vi "InitializeFile_useVariant.vi"(4 "Digitizer Info":T2, 5 "QDC Info":T2, 6 "TDC Info":T2, 7 "Scaler Info":T2, 8 "error in":errorcluster, 9 "Trigger Bit Descriptions":string[](array[string]), 10 "Thermocouple Location":string[](array[string]), 11 "File Path":path) -> (0 "error out":errorcluster, 3 "File Handle":T1 format="%.0x")   [LabVIEW 2014]
uses:
  <vilib>/addons/h5labview2/base/hid_t.ctl
  <vilib>/addons/h5labview2/file/H5Fmode.ctl
  DatasetNames.vi
  <vilib>/addons/h5labview2/base/lib_path.vi
  <vilib>/addons/h5labview2/base/H5Equery.vi
  <vilib>/addons/h5labview2/attrib/H5Awrite.llb/H5Awrite.xnode
  <vilib>/addons/h5labview2/file/H5F.lvlib
  <vilib>/addons/h5labview2/group/H5G.lvlib
  <vilib>/addons/h5labview2/dataset/H5D.lvlib
  <vilib>/addons/h5labview2/attrib/H5A.lvlib
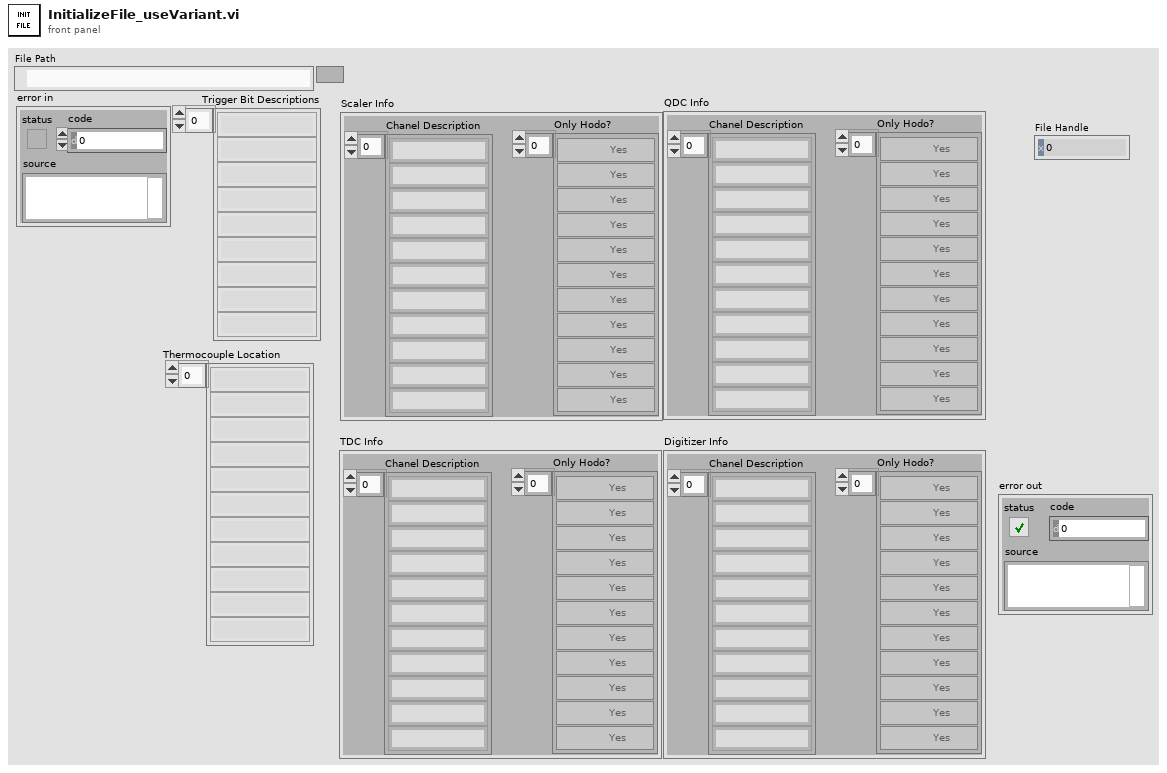
[diagram p1: front panel]
types:
  T1 = typedef "hid_t.ctl" = i32
  T2 = cluster{"Chanel Description":string[], "Only Hodo?":bool[]}
  T3 = typedef "H5F.lvlib/H5Fmode.ctl" = enum16{"read-only", "read-write", "overwrite", "create new", "open or create"}
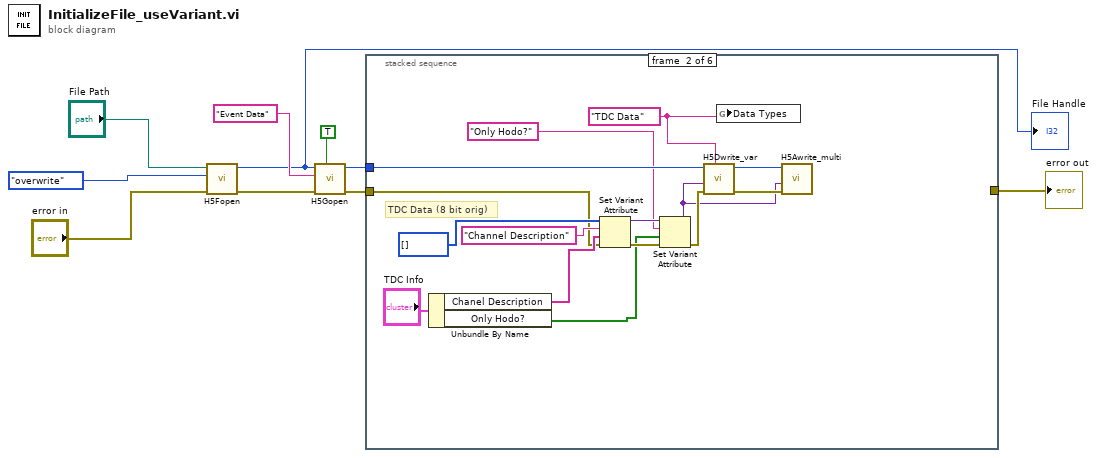
[diagram p0: block diagram]
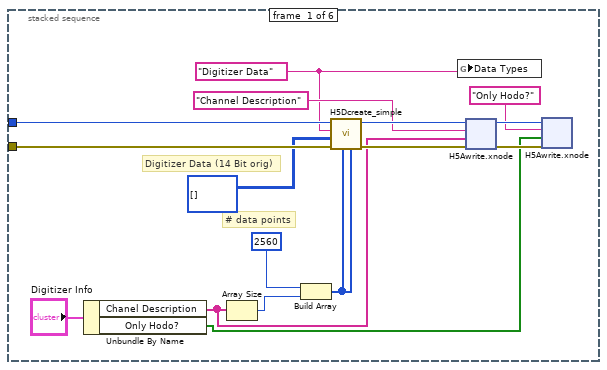
[diagram p2: hidden frame]
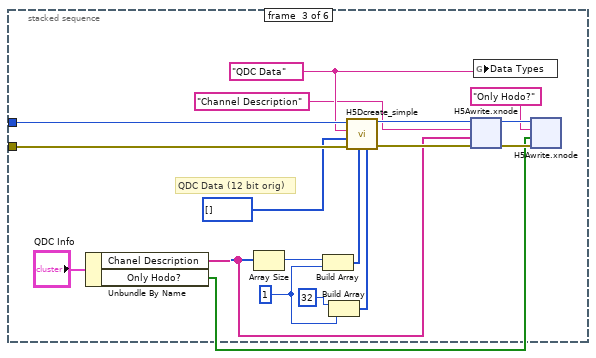
[diagram p3: hidden frame]
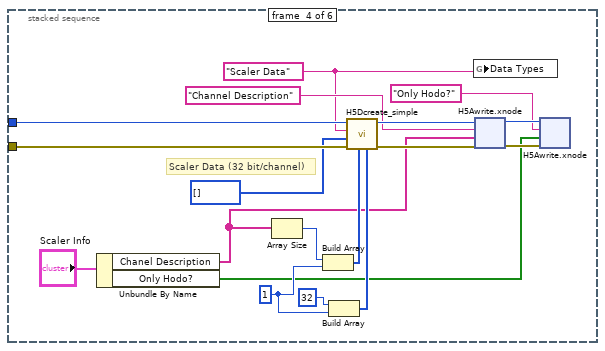
[diagram p4: hidden frame]
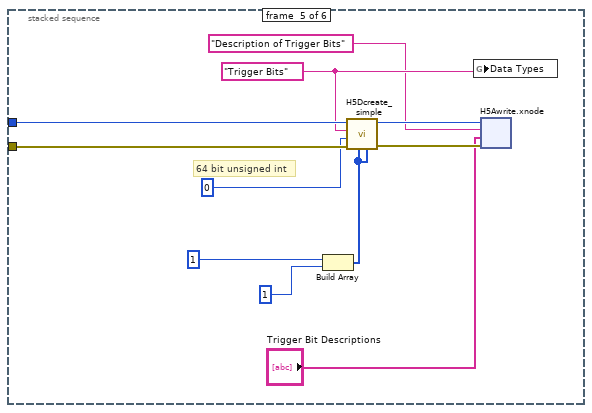
[diagram p5: hidden frame]
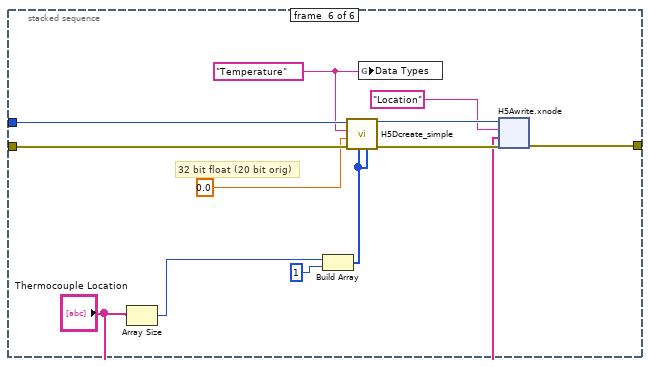
[diagram p6: hidden frame]
diagram:
  n1 = call <vilib>:"H5Fopen.vi"("error in (no error)"="error in", "mode (read-only)"=H5Fmode."overwrite", "path"="File Path") -> ("error out"=w7:errorcluster, "ref out"=w2:T1)  [unwired: 7 in]
  "File Handle" <- w2
  n2 = call <vilib>:"H5Gopen.vi"("create? (F)"=TRUE, "error in (no error)"=w7, "name"="Event Data", "ref in"=w2) -> ("error out"=w4:errorcluster, "group out"=w5:T1)  [unwired: 6 in]
  n3 = stacked-sequence {
    tunnel: w5 -> [w26 w77 w94 w148 w195 w225]
    tunnel: w4 -> [w25 w69 w95 w149 w196 w226]
    tunnel: [_ _ _ _ _ w219] -> w3
    frame #0 {
      w13 = "Digitizer Data" ("Combo Box")
      # "Digitizer Data (14 Bit orig)"
      # "# data points"
      n4 = Unbundle By Name("Digitizer Info") -> ("Chanel Description"=w16:string[], "Only Hodo?"=w11:bool[])
      n5 = Array Size(array=w16) -> (size(s)=w20:i32)
      n6 = Build Array(2560, w20) -> (w22:i32[])
      n7 = call <vilib>:"H5Dcreate_simple.vi"("max size"=w22, "initial size"=w22, "error in (no error)"=w25, "type in"=i16[][] [] ("Digitizer Data (14 Bit orig)"), "name"=w13, "ref in"=w26) -> ("error out"=w19:errorcluster, "dset out"=w18:T1)  [unwired: 4 in]
      n8 = global write "DatasetNames.vi" "Data Types"(w13) -> ()
      n9 = xnode "H5Awrite.xnode"("error in (no error)"=w19, "data"=w16, "attrib name"="Channel Description", "ref in"=w18) -> ("error out"=w15:errorcluster, "ref out"=w14:i32)  [unwired: 3 in, 1 out]
      n10 = xnode "H5Awrite.xnode"("error in (no error)"=w15, "data"=w11, "attrib name"="Only Hodo?", "ref in"=w14) -> ()  [unwired: 3 in, 3 out]
    }
    frame #1 {
      w75 = "TDC Data" ("Combo Box")
      # "TDC Data (8 bit orig)"
      n11 = Unbundle By Name("TDC Info") -> ("Chanel Description"=w72:string[], "Only Hodo?"=w67:bool[])
      n12 = Set Variant Attribute(Variant=i16[] [] ("TDC Data (8 bit orig)"), name="Channel Description" ("attrib name"), value=w72, error in=w69) -> (Variant out=w70:variant, error out=w71:errorcluster)  [unwired: 1 out]
      n13 = Set Variant Attribute(Variant=w70, name="Only Hodo?" ("attrib name"), value=w67, error in=w71) -> (Variant out=w63:variant, error out=w66:errorcluster)  [unwired: 1 out]
      n14 = call <vilib>:"H5Dwrite_var.vi"("dataset name"=w75, "error in (no error)"=w66, "data"=w63, "ref in"=w77) -> ("error out"=w64:errorcluster, "ref out"=w65:T1)  [unwired: 5 in, 1 out]
      n15 = global write "DatasetNames.vi" "Data Types"(w75) -> ()
      n16 = call <vilib>:"H5Awrite_multi.vi"("error in (no error)"=w64, "variant in"=w63, "ref in"=w65) -> ()  [unwired: 7 in, 2 out]
    }
    frame #2 {
      w91 = 1 ("element")
      w88 = "QDC Data" ("Combo Box")
      # "QDC Data (12 bit orig)"
      n17 = Unbundle By Name("QDC Info") -> ("Chanel Description"=w80:string[], "Only Hodo?"=w78:bool[])
      n18 = Array Size(array=w80) -> (size(s)=w81:i32)
      n19 = Build Array(w81, w91) -> (w92:i32[])
      n20 = Build Array(32 ("element"), w91) -> (w89:i32[])
      n21 = call <vilib>:"H5Dcreate_simple.vi"("max size"=w89, "initial size"=w92, "error in (no error)"=w95, "type in"=i16[] [] ("QDC Data (12 bit orig)"), "name"=w88, "ref in"=w94) -> ("error out"=w85:errorcluster, "dset out"=w87:T1)  [unwired: 4 in]
      n22 = xnode "H5Awrite.xnode"("error in (no error)"=w85, "data"=w80, "attrib name"="Channel Description", "ref in"=w87) -> ("error out"=w84:errorcluster, "ref out"=w83:i32)  [unwired: 3 in, 1 out]
      n23 = global write "DatasetNames.vi" "Data Types"(w88) -> ()
      n24 = xnode "H5Awrite.xnode"("error in (no error)"=w84, "data"=w78, "attrib name"="Only Hodo?", "ref in"=w83) -> ()  [unwired: 3 in, 3 out]
    }
    frame #3 {
      w145 = 1 ("element")
      w132 = "Scaler Data" ("Combo Box")
      # "Scaler Data (32 bit/channel)"
      n25 = Unbundle By Name("Scaler Info") -> ("Chanel Description"=w134:string[], "Only Hodo?"=w133:bool[])
      n26 = Array Size(array=w134) -> (size(s)=w136:i32)
      n27 = Build Array(w136, w145) -> (w146:i32[])
      n28 = Build Array(32 ("element"), w145) -> (w143:i32[])
      n29 = call <vilib>:"H5Dcreate_simple.vi"("max size"=w143, "initial size"=w146, "error in (no error)"=w149, "type in"=u32[] [] ("Scaler Data (32 bit/channel)"), "name"=w132, "ref in"=w148) -> ("error out"=w141:errorcluster, "dset out"=w142:T1)  [unwired: 4 in]
      n30 = global write "DatasetNames.vi" "Data Types"(w132) -> ()
      n31 = xnode "H5Awrite.xnode"("error in (no error)"=w141, "data"=w134, "attrib name"="Channel Description", "ref in"=w142) -> ("error out"=w139:errorcluster, "ref out"=w138:i32)  [unwired: 3 in, 1 out]
      n32 = xnode "H5Awrite.xnode"("error in (no error)"=w139, "data"=w133, "attrib name"="Only Hodo?", "ref in"=w138) -> ()  [unwired: 3 in, 3 out]
    }
    frame #4 {
      w189 = "Trigger Bits" ("Combo Box")
      # "64 bit unsigned int"
      n33 = Build Array(1 ("element"), 1 ("element")) -> (w191:i32[])
      n34 = call <vilib>:"H5Dcreate_simple.vi"("max size"=w191, "initial size"=w191, "error in (no error)"=w196, "type in"=u64 0, "name"=w189, "ref in"=w195) -> ("error out"=w187:errorcluster, "dset out"=w190:T1)  [unwired: 4 in]
      n35 = global write "DatasetNames.vi" "Data Types"(w189) -> ()
      n36 = xnode "H5Awrite.xnode"("error in (no error)"=w187, "data"="Trigger Bit Descriptions", "attrib name"="Description of Trigger Bits", "ref in"=w190) -> ()  [unwired: 3 in, 3 out]
    }
    frame #5 {
      w220 = "Temperature" ("Combo Box")
      # "32 bit float (20 bit orig)"
      n37 = Array Size(array="Thermocouple Location") -> (size(s)=w217:i32)
      n38 = Build Array(w217, 1 ("element")) -> (w215:i32[])
      n39 = call <vilib>:"H5Dcreate_simple.vi"("max size"=w215, "initial size"=w215, "error in (no error)"=w226, "type in"=sgl 0.0, "name"=w220, "ref in"=w225) -> ("error out"=w223:errorcluster, "dset out"=w222:T1)  [unwired: 4 in]
      n40 = global write "DatasetNames.vi" "Data Types"(w220) -> ()
      n41 = xnode "H5Awrite.xnode"("error in (no error)"=w223, "data"="Thermocouple Location", "attrib name"="Location", "ref in"=w222) -> ("error out"=w219:errorcluster)  [unwired: 3 in, 2 out]
    }
  }
  "error out" <- w3
